vi "Polynomial Evaluate.vi"(9 "Data":dbl, 10 "Coefficients":dbl[](array[numeric])) -> (1 "Results":dbl)   [LabVIEW 2020, in "VolatusData.lvlib" / "Scaling.lvclass"]
uses:
  VolatusData/DataProcessor/DataProcessor.lvclass/DataProcessor.ctl
  Scaling.lvclass
  Scaling.lvclass/Scaling.ctl
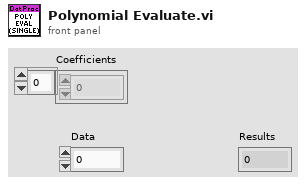
[diagram p1: front panel]
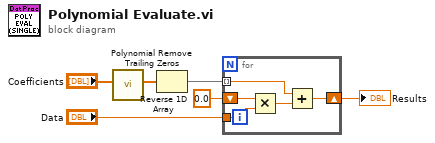
[diagram p0: block diagram]
diagram:
  n1 = call "Polynomial Remove Trailing Zeros.vi"("Coefficients"="Coefficients") -> ("Used Coefficients"=w5:dbl[])  [unwired: 10 in]
  n2 = Reverse 1D Array(array=w5) -> (reversed array=w4:dbl[])
  n3 = for {
    tunnel: w4 -> [w8] mode=indexing
    tunnel: "Data" -> [w10]
    shift-right: [w7] -> w2
    shift-left: 0.0 -> [w11]
    n4 = Multiply(x=w11, y=w10) -> (x*y=w9:dbl)
    n5 = Add(x=w8, y=w9) -> (x+y=w7:dbl)
  }
  "Results" <- w2
